vi "AOD Message Loop.vi"(8 "error in (no error)":errorcluster, 9 "Data Queue":refnum<queue>, 10 "Data Notifier":refnum<notifier>, 11 "Message Queues":T1) -> (0 "error out":errorcluster)   [LabVIEW 2015, in "AOD.lvlib"]
uses:
  AOD.lvlib
  support/Message Queue/All Message Queues.ctl
  support/Message Queue/Message Cluster.ctl
  AOD Configuration.ctl
  AOD State.ctl
  AOD Loop State.ctl
  <vilib>/DAQmx/write.llb/DAQmx Write (Analog 1D DBL NChan 1Samp).vi
  <vilib>/DAQmx/miscellaneous.llb/DAQmx Fill In Error Info.vi
  <vilib>/Utility/error.llb/Error Cluster From Error Code.vi
  <vilib>/ErrorRing/Error Ring.xnode
  support/Message Queue/Message Queue.lvlib
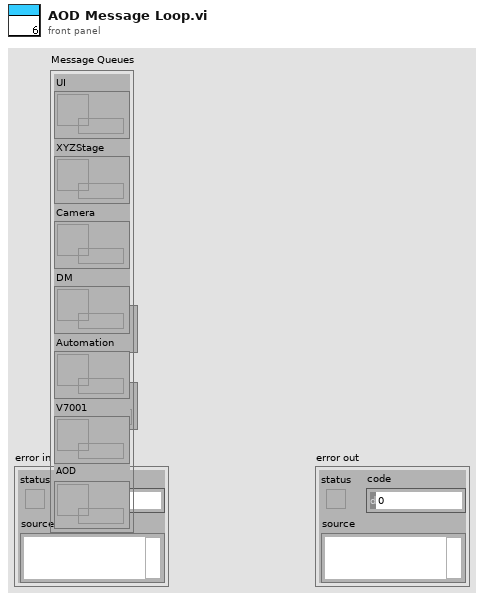
[diagram p1: front panel]
types:
  T1 = typedef "Message Queue.lvlib/All Message Queues.ctl" = cluster{"UI":refnum<queue>, "XYZStage":refnum<queue>, "Camera":refnum<queue>, "DM":refnum<queue>, "Automation":refnum<queue>, "V7001":refnum<queue>, "AOD":refnum<queue>}
  T2 = typedef "AOD.lvlib/AOD State.ctl" = cluster{"AOD State":T3, "daq task":refnum<k21>, "AOD Configuration":T4}
  T3 = typedef "AOD.lvlib/AOD Loop State.ctl" = enum16{"Idle", "Connected"}
  T4 = typedef "AOD.lvlib/AOD Configuration.ctl" = cluster{"Physical Channel":tag, "Maximum Value":dbl, "Minimum Value":dbl, "Update Rate":dbl}
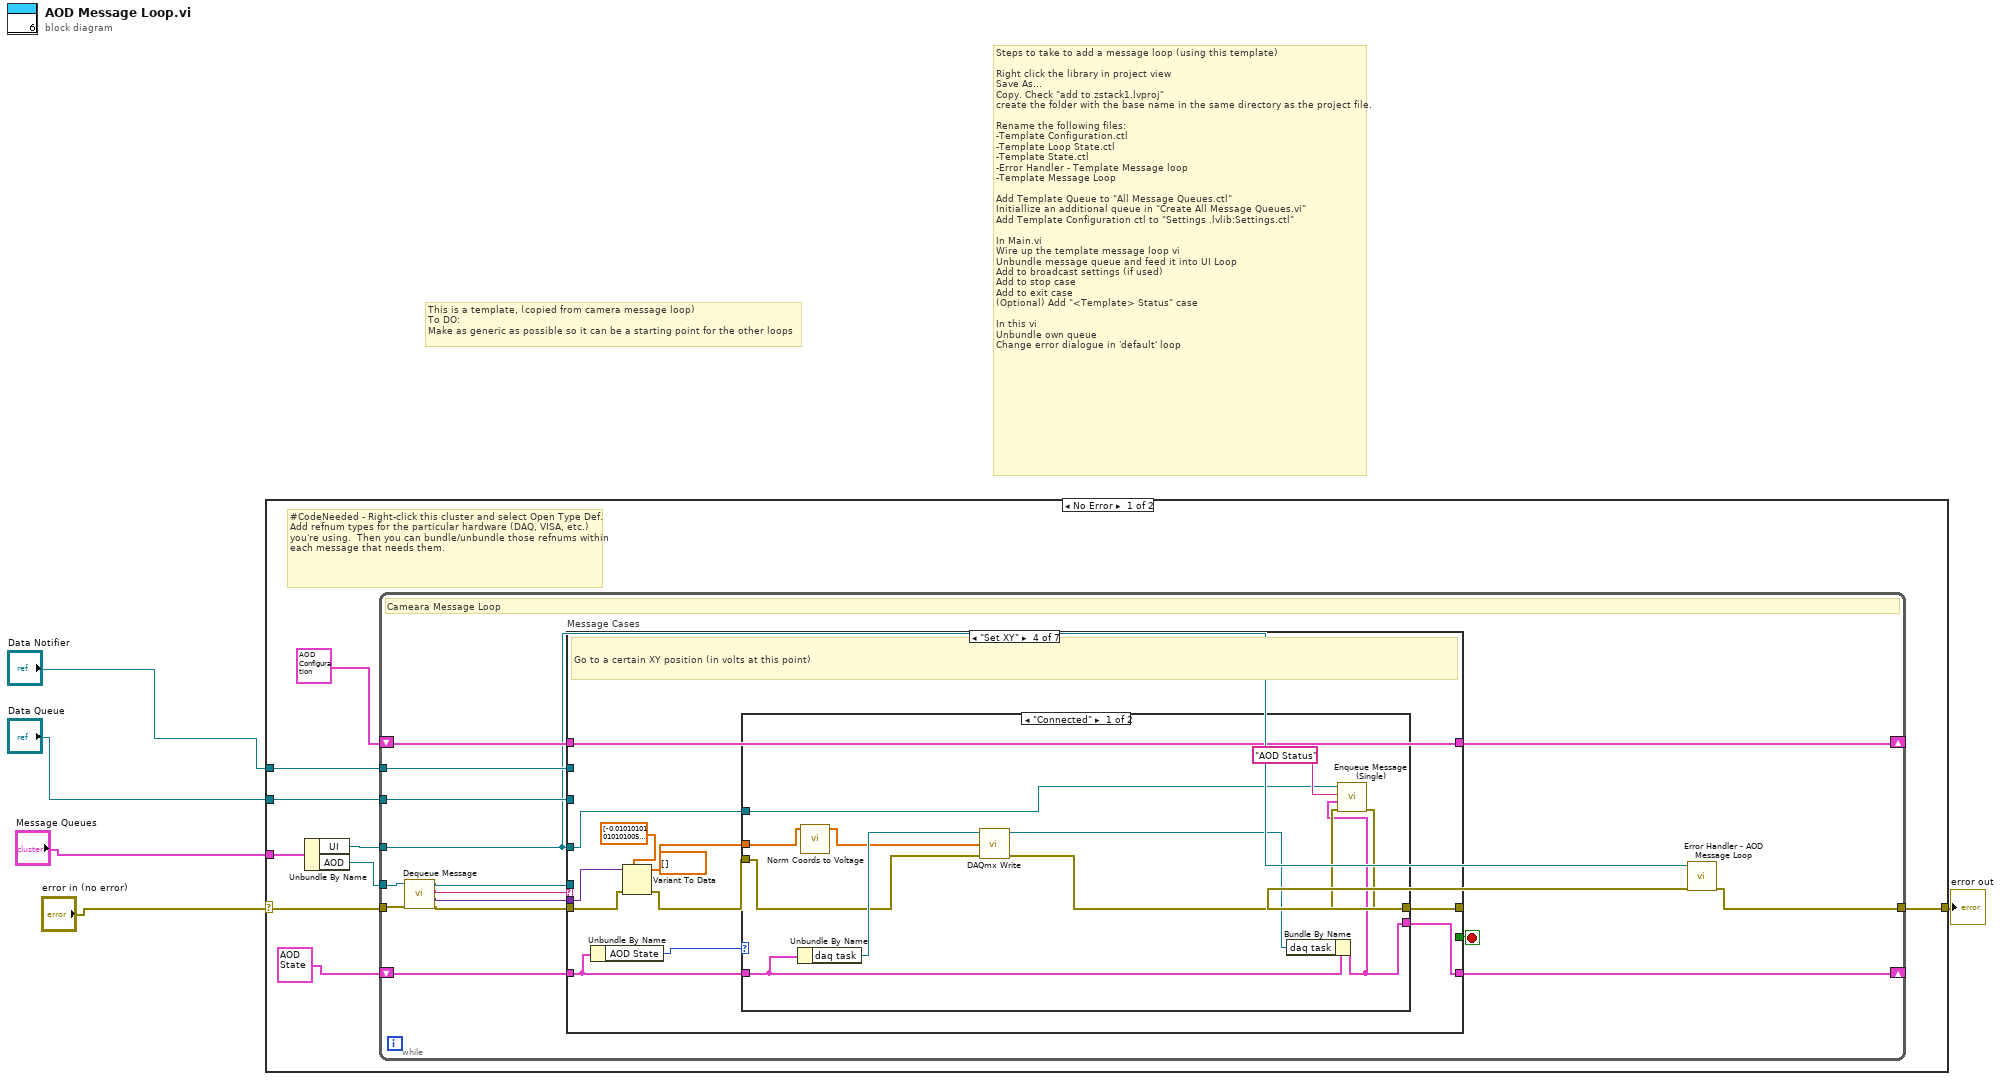
[diagram p0: block diagram]
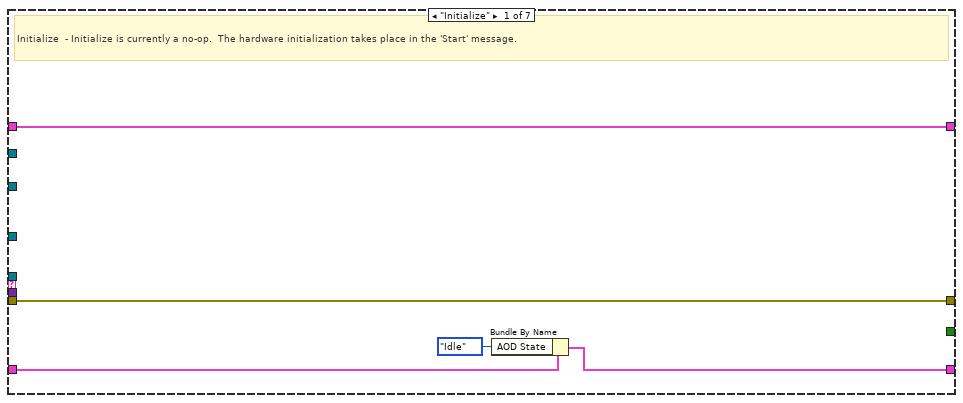
[diagram p2: hidden frame]
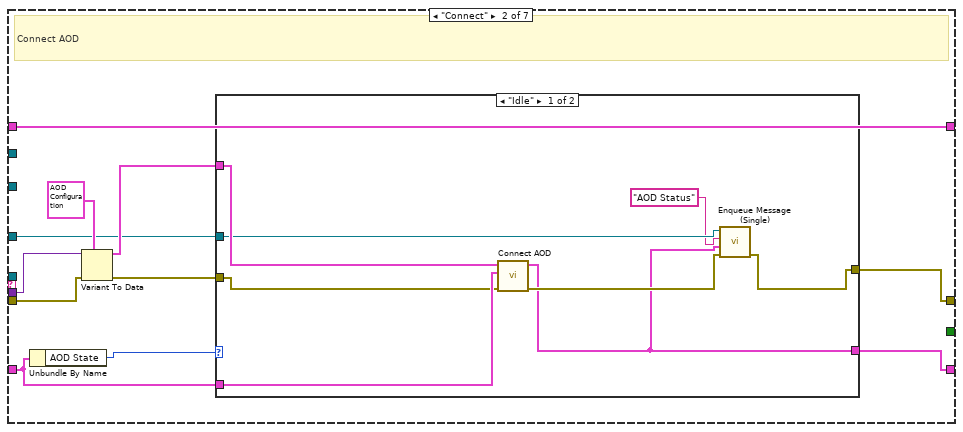
[diagram p3: hidden frame]
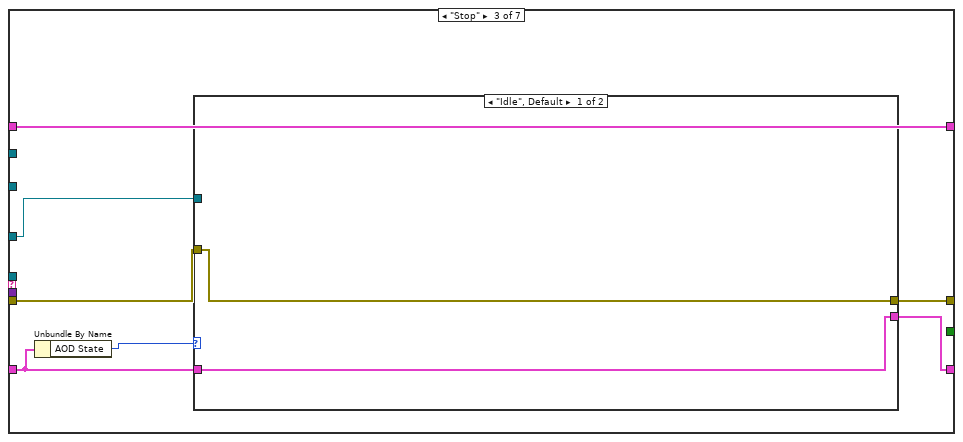
[diagram p5: hidden frame]
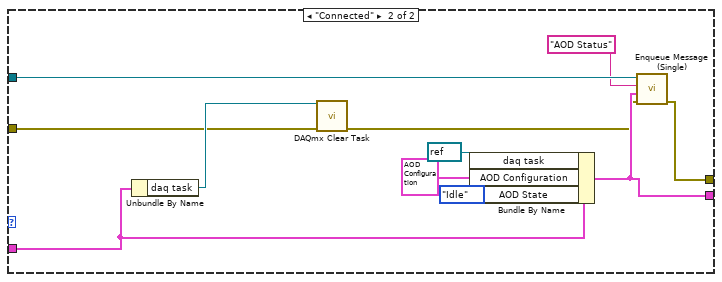
[diagram p6: hidden frame]
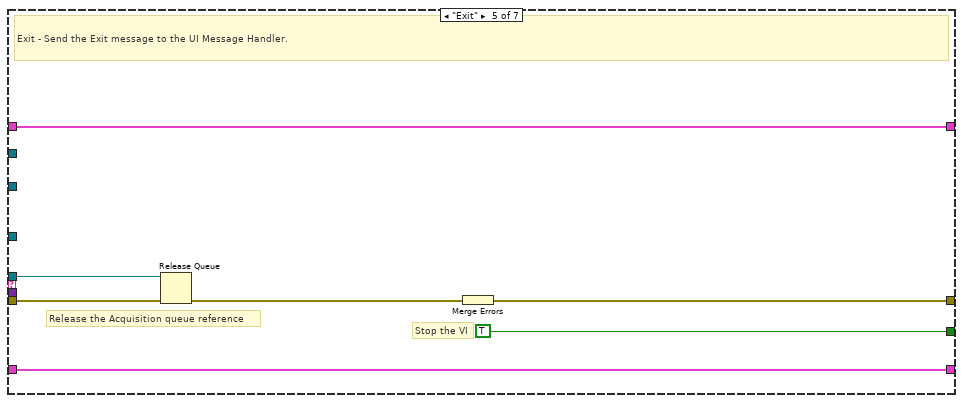
[diagram p8: hidden frame]
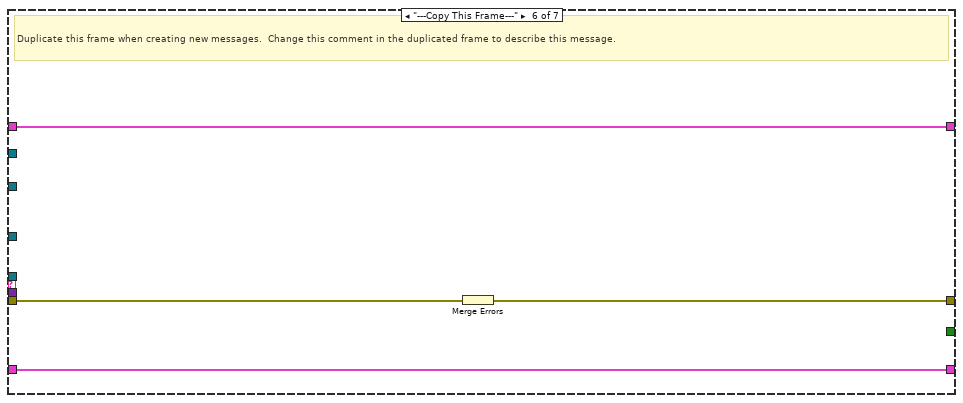
[diagram p9: hidden frame]
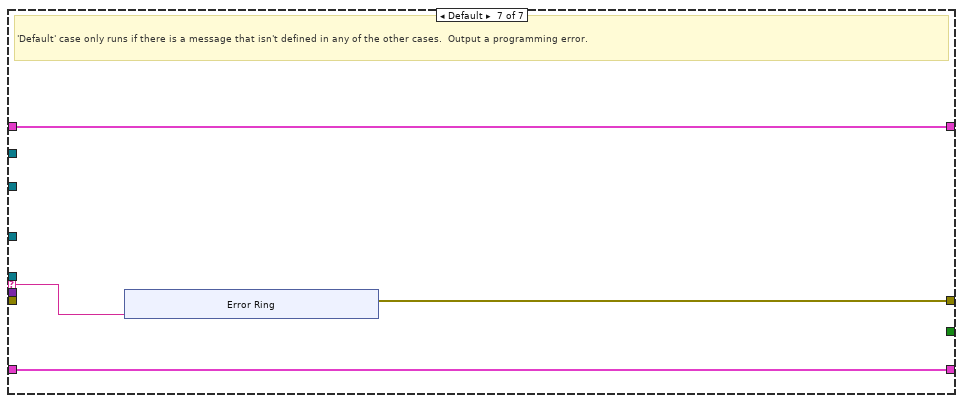
[diagram p10: hidden frame]
diagram:
  # "Steps to take to add a message loop (using this template)\n\nRight click the library in project view\nSave As...\nCopy. Check \"add to zstack1.lvproj\"\ncreate the folder with the base name in the same directory as the project file.\n\nRename the following files:\n-Template Configuration.ctl\n-Template Loop State.ctl\n-Template State.ctl\n-Error Handler - Template Message loop\n-Template Message Loop\n\nAdd Template Queue to \"All Message Queues.ctl\"\nInitiallize an additional queue in \"Create All Message Queues.vi\"\nAdd Template Configuration ctl to \"Settings .lvlib:Settings.ctl\"\n\nIn Main.vi\nWire up the template message loop vi\nUnbundle message queue and feed it into UI Loop\nAdd to broadcast settings (if used)\nAdd to stop case\nAdd to exit case\n(Optional) Add \"<Template> Status\" case\n\nIn this vi\nUnbundle own queue\nChange error dialogue in 'default' loop"
  # "This is a template, (copied from camera message loop)\nTo DO:\nMake as generic as possible so it can be a starting point for the other loops"
  n1 = case shown="No Error" "error in (no error)" {
    selector: "error in (no error)" -> [w11 w123]
    tunnel: "Message Queues" -> [w14 _]
    tunnel: [w12 w123] -> w5
    tunnel: "Data Notifier" -> [w9 _]
    tunnel: "Data Queue" -> [w8 _]
    frame No Error {
      # "#CodeNeeded - Right-click this cluster and select Open Type Def.  Add refnum types for the particular hardware (DAQ, VISA, etc.) you're using.  Then you can bundle/unbundle those refnums within each message that needs them."
      n2 = Unbundle By Name(w14) -> ("UI"=w10:refnum<queue>, "AOD"=w13:refnum<queue>)
      n3 = while {
        tunnel: w13 -> [w23]
        shift-right: [w29] -> _
        shift-left: T4 {"Physical Channel"="Dev1/ao0:1", "Maximum Value"=0.0, "Minimum Value"=1.0, "Update Rate"=192000.0} ("Hardware Configuration") -> [w30]
        tunnel: w10 -> [w15]
        tunnel: w9 -> [w27]
        tunnel: w8 -> [w26]
        shift-right: [w24] -> _
        shift-left: T2 {"AOD State"=enum."Idle", "daq task"="", "AOD Configuration"={"Physical Channel"="Dev1/ao0:1", "Maximum Value"=10.0, "Minimum Value"=1.0, "Update Rate"=192000.0}} ("Cluster") -> [w25]
        tunnel: w11 -> [w22]
        tunnel: [w17] -> w12
        stop <- w28 stop-if-true
        # "Cameara Message Loop"
        n4 = call "Dequeue Message.vi"("error in (no error)"=w22, "Message Queue"=w23) -> ("error out"=w18:errorcluster, "Message Data"=w19:variant, "Message"=w20:string, "dup Message Queue"=w21:refnum<queue>)  [unwired: 6 in]
        n5 = case "Message Cases" shown="\"Set XY\"" w20 {
          selector: w20 -> [_ _ _ _ _ _ w112]
          tunnel: w21 -> [_ _ _ _ w102 _ _]
          tunnel: w18 -> [w35 w43 w60 w80 w104 w111 _]
          tunnel: [w35 w37 w57 w82 w106 w109 w113] -> w16
          tunnel: w30 -> [w34 w46 w63 w87 w105 w110 w115]
          tunnel: [w34 w46 w63 w87 w105 w110 w115] -> w29
          tunnel: [_ _ _ _ TRUE _ _] -> w28
          tunnel: w19 -> [_ w44 _ w81 _ _ _]
          tunnel: w15 -> [_ w36 w58 w83 _ _ _]
          tunnel: w27 -> [_ _ _ _ _ _ _]
          tunnel: w26 -> [_ _ _ _ _ _ _]
          tunnel: w25 -> [w33 w39 w61 w85 w101 w108 w114]
          tunnel: [w32 w40 w59 w84 w101 w108 w114] -> w24
          frame "Initialize" {
            # "Initialize  - Initialize is currently a no-op.  The hardware initialization takes place in the 'Start' message."
            n6 = Bundle By Name(cluster=w33, "AOD State"=AOD_Loop_State."Idle") -> (w32:T2)
          }
          frame "Connect" {
            # "Connect AOD"
            n7 = Unbundle By Name(w39) -> ("AOD State"=w45:T3)
            n8 = Variant To Data(error in=w43, type=T4 {"Physical Channel"="Dev1/ao0:1", "Maximum Value"=10.0, "Minimum Value"=1.0, "Update Rate"=192000.0} ("AOD Configuration"), Variant=w44) -> (data=w41:T4, error out=w38:errorcluster)
            n9 = case shown="\"Idle\"" w45 {
              tunnel: w41 -> [w54 _]
              tunnel: [w47 w55] -> w40
              tunnel: w39 -> [w53 w55]
              tunnel: w38 -> [w52 w56]
              tunnel: [w49 w56] -> w37
              tunnel: w36 -> [w51 _]
              frame "Idle" {
                n10 = call "Connect AOD.vi"("error in (no error)"=w52, "AOD Status In"=w53, "AOD Configuration"=w54) -> ("error out"=w50:errorcluster, "AOD Status Out"=w47:T2)  [unwired: 7 in]
                n11 = call "Enqueue Message (Single).vi"("error in (no error)"=w50, "Message Data"=w47, "Message"="AOD Status", "Message Queue"=w51) -> ("error out"=w49:errorcluster)  [unwired: 6 in, 1 out]
              }
              frame "Connected", Default {
              }
            }
          }
          frame "Stop" {
            n12 = Unbundle By Name(w61) -> ("AOD State"=w62:T3)
            n13 = case shown="\"Idle\", Default" w62 {
              tunnel: w61 -> [w64 w74]
              tunnel: w60 -> [w65 w75]
              tunnel: [w64 w68] -> w59
              tunnel: w58 -> [_ w70]
              tunnel: [w65 w66] -> w57
              frame "Idle", Default {
              }
              frame "Connected" {
                n14 = Unbundle By Name(w74) -> ("daq task"=w76:refnum<k21>)
                n15 = call <vilib>:"DAQmx Clear Task.vi"("task in"=w76, "error in"=w75) -> ("error out"=w67:errorcluster)  [unwired: 13 in]
                n16 = Bundle By Name(cluster=w74, "daq task"=refnum<k21> refnum, "AOD Configuration"=T4 {"Physical Channel"="Dev1/ao0:1", "Maximum Value"=10.0, "Minimum Value"=1.0, "Update Rate"=192000.0}, "AOD State"=AOD_Loop_State."Idle") -> (w68:T2)
                n17 = call "Enqueue Message (Single).vi"("error in (no error)"=w67, "Message Data"=w68, "Message"="AOD Status", "Message Queue"=w70) -> ("error out"=w66:errorcluster)  [unwired: 6 in, 1 out]
              }
            }
          }
          frame "Set XY" {
            (unwired) dbl[] [] ("data")
            # "Go to a certain XY position (in volts at this point)"
            n18 = Unbundle By Name(w85) -> ("AOD State"=w86:T3)
            n19 = Variant To Data(error in=w80, type=dbl[] [-0.010101010101010055, 0.0010101010101010027, 0.0, 0.0, 0.0, -0.06565656565656566, 0.0, 0.0, 0.043434343434343436, 0.0, 0.0, 0.0, 0.0, 0.0, 0.0] ("X,Y"), Variant=w81) -> (data=w77:dbl[], error out=w79:errorcluster)
            n20 = case shown="\"Connected\"" w86 {
              tunnel: w85 -> [w96 w99]
              tunnel: w79 -> [w97 w100]
              tunnel: [w91 w99] -> w84
              tunnel: w83 -> [w90 _]
              tunnel: [w92 w100] -> w82
              tunnel: w77 -> [w89 _]
              frame "Connected" {
                n21 = Unbundle By Name(w96) -> ("daq task"=w98:refnum<k21>)
                n22 = call "Norm Coords to Voltage.vi"("coords in"=w89) -> ("voltage out"=w88:dbl[])  [unwired: 10 in]
                n23 = call-poly <vilib>:"DAQmx Write.vi"("task/channels in"=w98, "data"=w88, "error in"=w97) -> ("task out"=w95:refnum<k21>, "error out"=w93:errorcluster)  [unwired: 10 in, 1 out]
                n24 = Bundle By Name(cluster=w96, "daq task"=w95) -> (w91:T2)
                n25 = call "Enqueue Message (Single).vi"("error in (no error)"=w93, "Message Data"=w91, "Message"="AOD Status", "Message Queue"=w90) -> ("error out"=w92:errorcluster)  [unwired: 6 in, 1 out]
              }
              frame "Idle" {
              }
            }
          }
          frame "Exit" {
            # "Release the Acquisition queue reference"
            # "Stop the VI"
            # "Exit - Send the Exit message to the UI Message Handler."
            n26 = Release Queue(queue=w102, error in (no error)=w104) -> (error out=w103:errorcluster)  [unwired: 1 in, 2 out]
            n27 = Merge Errors(w103) -> (w106:errorcluster)
          }
          frame "---Copy This Frame---" {
            # "Duplicate this frame when creating new messages.  Change this comment in the duplicated frame to describe this message."
            n28 = Merge Errors(w111) -> (w109:errorcluster)
          }
          frame Default {
            # "'Default' case only runs if there is a message that isn't defined in any of the other cases.  Output a programming error."
            n29 = xnode "Error Ring"("parameter 0"=w112) -> ("error out"=w113:errorcluster)
          }
        }
        n30 = call "Error Handler - AOD Message Loop.vi"("error in (no error)"=w16, "Message Queue"=w15) -> ("dup error in"=w17:errorcluster)  [unwired: 8 in, 1 out]
      }
    }
    frame Error {
    }
  }
  "error out" <- w5
